vi "Read Voltage.vi"(6 "에러 입력":cluster{"상태":bool, "코드":i32, "소스":string}) -> (0 "에러 출력":cluster{"상태":bool, "코드":i32, "소스":string}, 3 "전압":dbl)   [LabVIEW 2015]
doc: "이 VI는 LabVIEW Core 1 및 2 교육과정에서 사용됩니다.\n\n이 VI는 DAQ 보드에서 전압 값 읽기를 시뮬레이션합니다. 이 교육과정의 모든 온도 읽기 관련 연습문제에서 [DAQ 어시스턴트] 익스프레스 VI 대신 이 VI를 사용하십시오. 이 VI는 모든 (데모) 연습문제에서 SubVI로 사용됩니다."
panel:
  # "이 VI는 디바이스 1, 채널 0의 전압을 읽는 VI의 데모 버전입니다.  값은 100으로 스케일되어 온도값을 나타낼 수 있습니다."
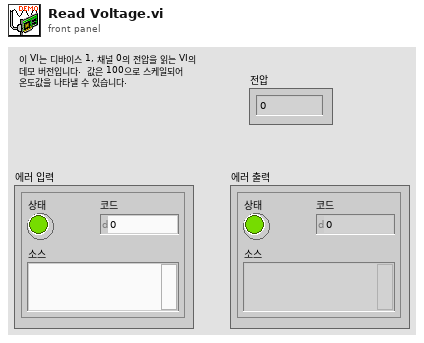
[diagram p1: front panel]
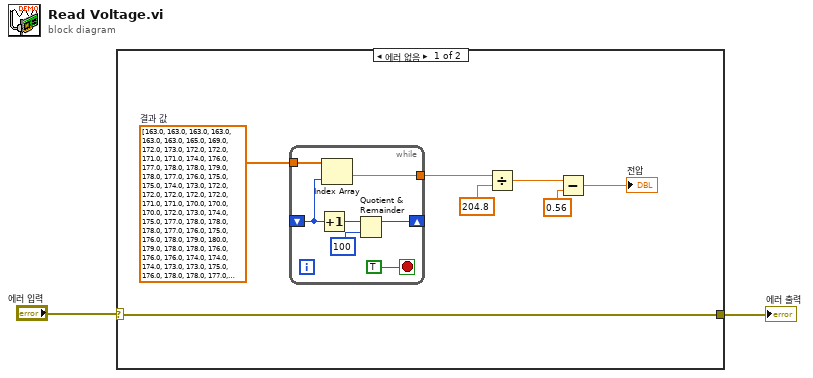
[diagram p0: block diagram]
diagram:
  n1 = case shown="에러 없음" "에러 입력" {
    selector: "에러 입력" -> [w5 w17]
    tunnel: [w5 w17] -> w2
    frame No Error {
      w3 = dbl[] [163.0, 163.0, 163.0, 163.0, 163.0, 163.0, 165.0, 169.0, 172.0, 173.0, 172.0, 172.0, 171.0, 171.0, 174.0, 176.0, 177.0, 178.0, 178.0, 179.0, 178.0, 177.0, 176.0, 175.0, 175.0, 174.0, 173.0, 172.0, 172.0, 172.0, 172.0, 172.0, 171.0, 171.0, 170.0, 170.0, 170.0, 172.0, 173.0, 174.0, 175.0, 177.0, 178.0, 178.0, 178.0, 177.0, 176.0, 175.0, 176.0, 178.0, 179.0, 180.0, 179.0, 178.0, 178.0, 176.0, 176.0, 176.0, 174.0, 174.0, 174.0, 173.0, 173.0, 175.0, 176.0, 178.0, 178.0, 177.0, 176.0, 175.0, 175.0, 174.0, 174.0, 173.0, 173.0, 172.0, 172.0, 171.0, 171.0, 170.0, 170.0, 170.0, 170.0, 170.0, 170.0, 170.0, 169.0, 166.0, 167.0, 169.0, 170.0, 169.0, 168.0, 168.0, 168.0, 168.0, 167.0, 167.0, 167.0, 167.0]  # 결과 값
      n2 = while {
        tunnel: w3 -> [w11]
        tunnel: [w12] -> w8
        shift-left: _ -> [w16]
        shift-right: [w13] -> _
        stop <- TRUE stop-if-true
        n3 = Increment(x=w16) -> (x+1=w15:i32)
        n4 = Index Array(array=w11, index=w16) -> (element=w12:dbl)
        n5 = Quotient & Remainder(x=w15, y=100) -> (x-y*floor(x/y)=w13:i32)  [unwired: 1 out]
      }
      n6 = Divide(x=w8, y=204.8) -> (x/y=w7:dbl)
      n7 = Subtract(x=w7, y=0.56) -> (x-y=→"전압":dbl)
    }
    frame Error {
    }
  }
  "에러 출력" <- w2
